vi "DraggingDresser.vi"() -> ()   [LabVIEW 2015]
panel:
  out "Force":dbl[](array[numeric])
  out "Angle for Minimum Force":i32 format="%.1f"
  in  "Coefficient of Kinetic Friction":dbl format="%.1f"
  out "Waveform Graph":dbl[](graph)
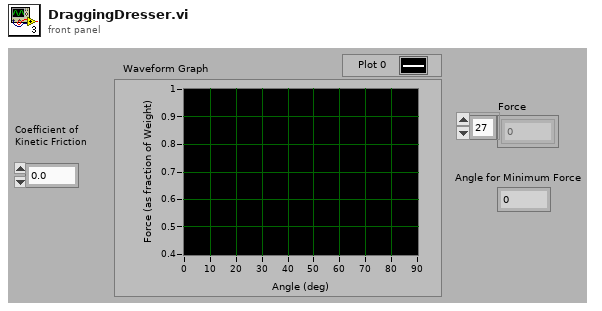
[diagram p1: front panel]
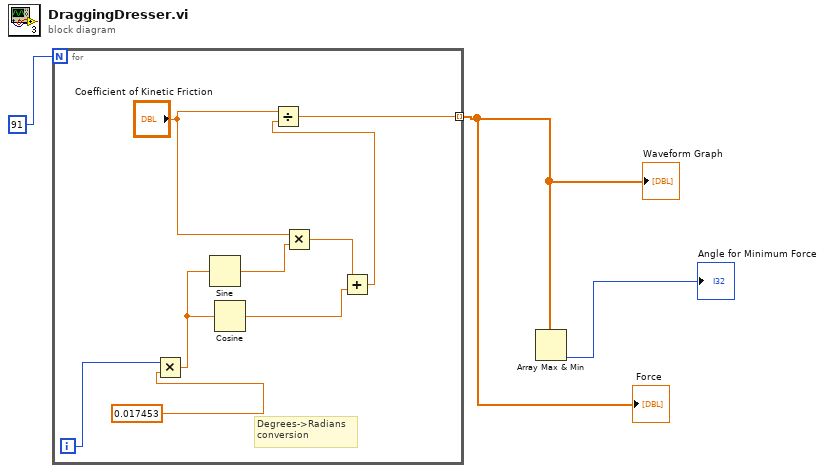
[diagram p0: block diagram]
diagram:
  n1 = for {
    N: 91 -> [_]
    tunnel: [w5] -> w1 mode=indexing
    i -> [w4]
    # "Degrees->Radians \nconversion"
    n2 = Multiply(x=w4, y=0.017453) -> (x*y=w11:dbl)
    n3 = Sine(x=w11) -> (sin(x)=w8:dbl)
    n4 = Cosine(x=w11) -> (cos(x)=w10:dbl)
    n5 = Multiply(x="Coefficient of Kinetic Friction", y=w8) -> (x*y=w7:dbl)
    n6 = Add(x=w7, y=w10) -> (x+y=w6:dbl)
    n7 = Divide(x="Coefficient of Kinetic Friction", y=w6) -> (x/y=w5:dbl)
  }
  "Waveform Graph" <- w1
  "Force" <- w1
  n8 = Array Max & Min(array=w1) -> (min index (indices)=→"Angle for Minimum Force":i32)  [unwired: 3 out]
